vi "Adjust Splitter.vi"(8 "error in":errorcluster, 9 "Show":bool, 10 "Splitter Info":T1, 11 "Prime Panel in":refnum<class "Prime Panel.lvclass">) -> (0 "error out":errorcluster, 3 "Prime Panel out":refnum<class "Prime Panel.lvclass">)   [LabVIEW 2019, in "Prime Panel.lvlib" / "Prime Panel.lvclass"]
doc: "This override is here so child classes can act on a show/hide event.\nPrime panel does not adjust splitters"
uses:
  Project/Prime Panel.lvclass
  builds/Engine/Engine.lvlibp/Project/Engine.lvclass
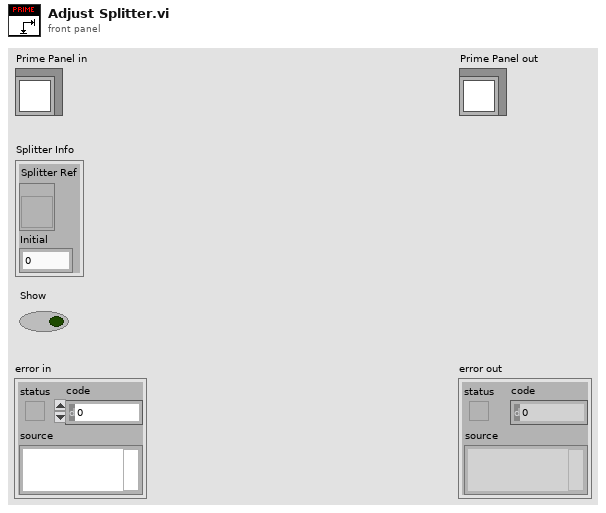
[diagram p1: front panel]
types:
  T1 = cluster{"Splitter Ref":refnum<vi>, "Initial":i32}
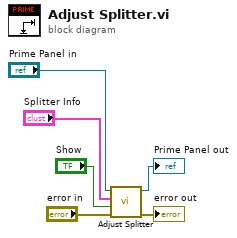
[diagram p0: block diagram]
diagram:
  n1 = call-parent "Adjust Splitter.vi"("error in"="error in", "Show"="Show", "Splitter Info"="Splitter Info", "Engine in"="Prime Panel in") -> ("error out"=→"error out":errorcluster, "Engine out"=→"Prime Panel out":refnum<class "Prime Panel.lvclass">)  [unwired: 6 in]
